vi "(SubVI) Acquire Sinewave True Amplitude A by using Waveform WriteRead_YCC.vi"(5 "f_drive (Hz)":dbl=32.0, 6 "Amplitude, A (nm)":dbl=500.0, 7 "Axis  (Enum)":enum16{"x", "y", "z"}(ring)) -> (1 "True f_drive (Hz)":dbl, 2 "True Amplitude, A (nm)":dbl)   [LabVIEW 2014]
uses:
  Main-Stage-Based/(Global) Current handle and LaserPower_YCC.vi
  <vilib>/gmath/NumericalOptimization/Nonlinear Curve Fit LM formula string.vi
  <vilib>/Utility/file.llb/Write To Spreadsheet File (DBL).vi
  <vilib>/gmath/NI_Gmath.lvlib
panel:
  out "size(s) 2":i32
  out "size(s)":i32
  out "Total Need time (s)":dbl format="%.5f"
  in  "Tab Control":enum32{"Command", "True Output", "Fitting"}(tab)
  out "Write XY Graph 2":cluster{dbl[], "Data Array Out to read":dbl[]}(graph)
  out "Read XY Graph":cluster{dbl[], "Data Array Out to read":dbl[]}(graph)
  out "Read XY Graph 2":cluster{dbl[], "Data Array Out to read":dbl[]}[](graph)
  out "best nonlinear fit for cut position":dbl[](array[numeric])
  in  "Save?":bool
  out "A scaling":dbl
  out "Axis":i32
  out "appended array":dbl[](array[numeric])
  out "Real Current Commanded position (um)":dbl format="%0.5f"
  out "Cut-position array":dbl[](array[numeric])
  out "Cut-Time array":dbl[](array[numeric])
  out "Position Array (um)":dbl[](array[numeric])
  out "Time Array (s)":dbl[](array[numeric])
  out "Sampling Rate (Hz)":dbl
  out "best fit parameters":dbl[](array[numeric])
  out "Read True Position Array (um)":dbl[](array[numeric]) format="%.2f"
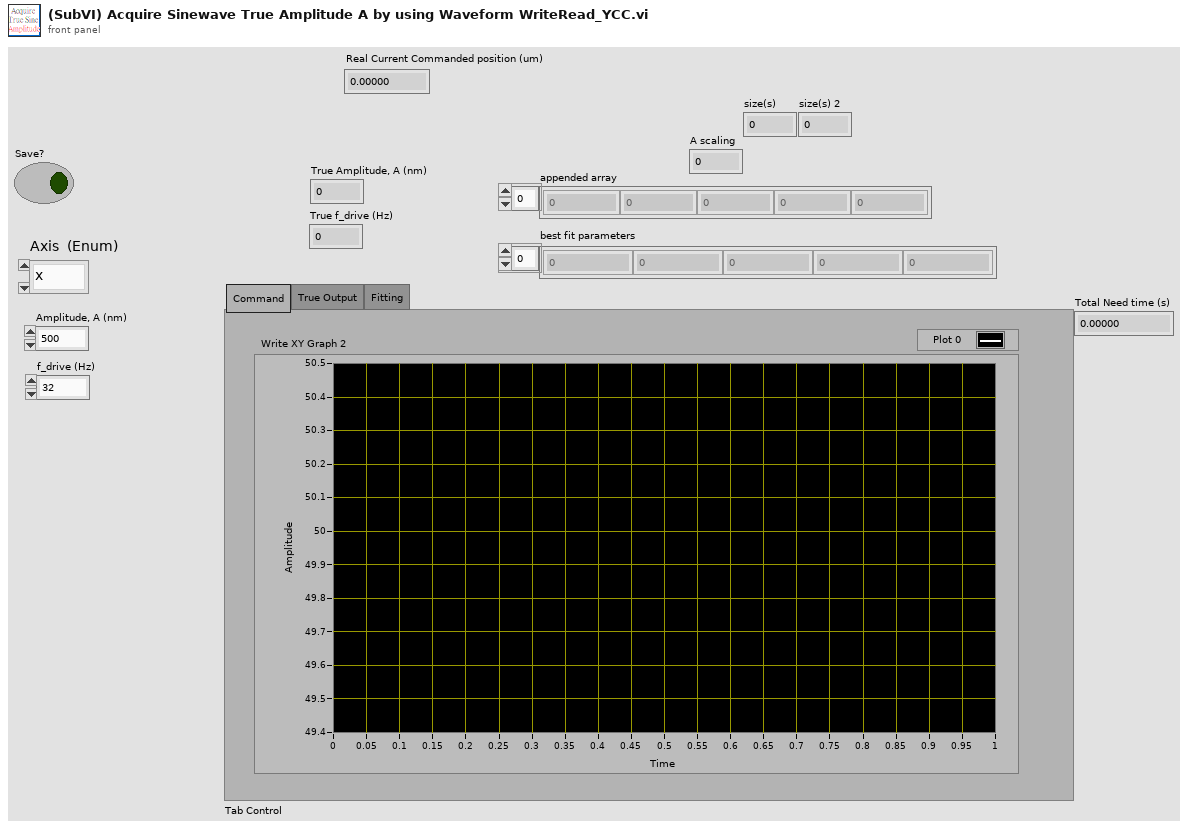
[diagram p1: front panel]
types:
  T1 = enum16{"50 Hz", "60 Hz", "100 Hz", "500 Hz", "1000 Hz", "2000 Hz", "3750 Hz"}
  T2 = cluster{"model":string, "Parameters":string[], "x":string}
  T3 = cluster{"Time Array (s)":dbl[], "Position Array (um)":dbl[]}
  T4 = cluster{"Cut-Time array":dbl[], "best nonlinear fit":dbl[]}
  T5 = cluster{"Cut-Time array":dbl[], "Cut-position array":dbl[]}
  T6 = cluster{"Cut-Time array":dbl[], "Cut-position array":dbl[]}[]
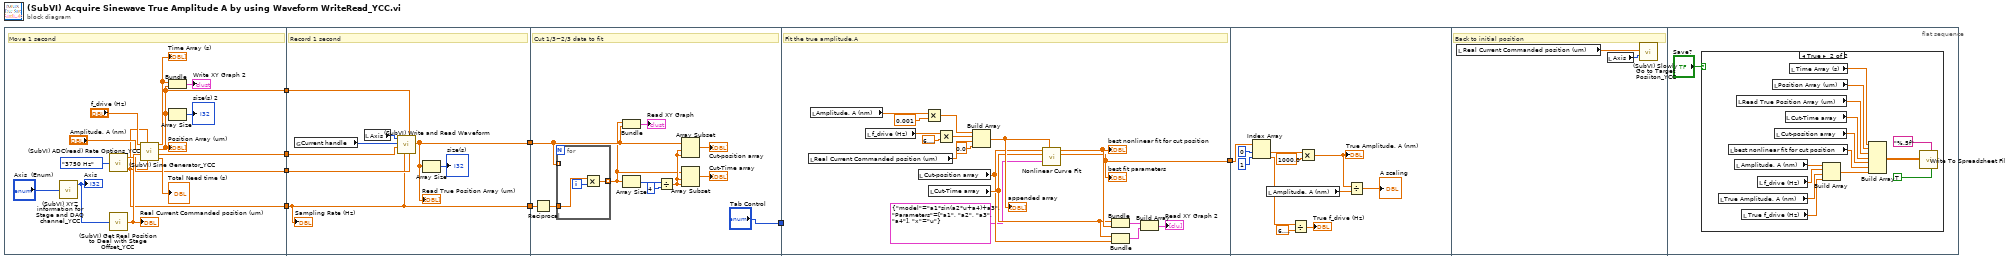
[diagram p0: block diagram]
diagram:
  n1 = flat-sequence {
    tunnel: [w17] -> w8
    tunnel: [w13] -> w7
    tunnel: [w10] -> w3
    tunnel: [w9] -> w2
    tunnel: w8 -> [w28]
    tunnel: w7 -> [w27]
    tunnel: [w26] -> w6
    tunnel: [w23] -> w4
    tunnel: w3 -> [w24]
    tunnel: w2 -> [w23]
    tunnel: w6 -> [w35]
    tunnel: w4 -> [w34]
    tunnel: ["Tab Control"] -> w1
    tunnel: [w54] -> w5
    tunnel: w1 -> [_]
    tunnel: w5 -> [w72]
    frame #0 {
      # "Move 1 second"
      n2 = call "(SubVI) XYZ information for Stage and DAQ channel_YCC.vi"("Axis  (Enum)"="Axis  (Enum)") -> ("Axis"=w15:i32)  [unwired: 3 in, 1 out]
      "Axis" <- w15
      n3 = call "(SubVI) ADC(read) Rate Options_YCC.vi"("ADC Rate for 20bit (ms)"=T1."3750 Hz") -> ("Sampling Rate for reading (Hz)"=w9:dbl, "waiting code for Reading (20bits)"=w10:dbl)  [unwired: 3 in]
      n4 = call "(SubVI) Get Real Position to Deal with Stage Offset_YCC.vi"("Axis"=w15) -> ("Real Current Commanded position (um)"=w20:dbl)  [unwired: 3 in, 1 out]
      "Real Current Commanded position (um)" <- w20
      n5 = call "(SubVI) Sine Generator_YCC.vi"("Points to be generated"=w9, "fs (Hz)"=w9, "initial position (um)"=w20, "Amplitude, A (nm)"="Amplitude, A (nm)", "f_drive (Hz)"="f_drive (Hz)") -> ("Total Need time (s)"=→"Total Need time (s)":dbl, "waiting time (to write) (ms)"=w17:dbl, "Position Array (um)"=w13:dbl[], "Time Array (s)"=w19:dbl[])  [unwired: 1 in]
      "Time Array (s)" <- w19
      "Position Array (um)" <- w13
      n6 = Bundle("Time Array (s)"=w19, "Position Array (um)"=w13) -> (→"Write XY Graph 2":T3)  [unwired: 1 in]
      n7 = Array Size(array=w13) -> (size(s)=→"size(s) 2":i32)
    }
    frame #1 {
      # "Record 1 second"
      n8 = global read "(Global) Current handle and LaserPower_YCC.vi" "Current handle"() -> (w30:i32)
      n9 = local read "Axis"() -> (w29:i32)
      n10 = call "(SubVI) Write and Read Waveform.vi"("ADC Rate (Read)(ms)"=w24, "Data Array In to write"=w27, "Number of Positions to Read"=w23, "DAC Rate (Write) (ms)"=w28, "handle"=w30, "Axis"=w29) -> ("Data Array Out to read"=w26:dbl[])  [unwired: 5 in]
      "Read True Position Array (um)" <- w26
      n11 = Array Size(array=w26) -> (size(s)=→"size(s)":i32)
      "Sampling Rate (Hz)" <- w23
    }
    frame #2 {
      # "Cut 1/3~2/3 data to fit"
      n12 = Reciprocal(x=w34) -> (1/x=w33:dbl)
      n13 = for {
        tunnel: w35 -> [_] mode=indexing
        tunnel: w33 -> [w43]
        tunnel: [w42] -> w32 mode=indexing
        i -> [w44]
        n14 = Multiply(x=w43, y=w44) -> (x*y=w42:dbl)
      }
      n15 = Bundle(w32, "Data Array Out to read"=w35) -> (→"Read XY Graph":cluster{dbl[], "Data Array Out to read":dbl[]})  [unwired: 1 in]
      n16 = Array Size(array=w32) -> (size(s)=w40:i32)
      n17 = Divide(x=w40, y=4) -> (x/y=w38:dbl)
      n18 = Array Subset(array=w35, index=w38, length=w38) -> (→"Cut-position array":dbl[])
      n19 = Array Subset(array=w32, index=w38, length=w38) -> (→"Cut-Time array":dbl[])
    }
    frame #3 {
      # "Fit the true amplitude,A"
      n20 = local read "Real Current Commanded position (um)"() -> (w57:dbl)
      n21 = local read "Amplitude, A (nm)"() -> (w53:dbl)
      n22 = local read "f_drive (Hz)"() -> (w47:dbl)
      n23 = local read "Cut-position array"() -> (w49:dbl[])
      n24 = Multiply(x=w53, y=0.001) -> (x*y=w51:dbl)
      n25 = local read "Cut-Time array"() -> (w50:dbl[])
      n26 = Multiply(x=w47, y=6.283185307179586) -> (x*y=w45:dbl)
      n27 = Build Array(w51, w45, w57, 0.0 ("element")) -> (w55:dbl[])
      "appended array" <- w55
      n28 = call-poly <vilib>:"Nonlinear Curve Fit.vi"("Y"=w49, "initial parameters"=w55, "X"=w50, "model description"=T2 {"model"="a1*sin(a2*u+a4)+a3", "Parameters"=["a1", "a2", "a3", "a4"], "x"="u"}) -> ("best nonlinear fit"=w60:dbl[], "best fit parameters"=w54:dbl[])  [unwired: 7 in, 3 out]
      "best fit parameters" <- w54
      "best nonlinear fit for cut position" <- w60
      n29 = Bundle("Cut-Time array"=w50, "best nonlinear fit"=w60) -> (w59:T4)  [unwired: 1 in]
      n30 = Bundle("Cut-Time array"=w50, "Cut-position array"=w49) -> (w58:T5)  [unwired: 1 in]
      n31 = Build Array(w59, w58) -> (→"Read XY Graph 2":T6)
    }
    frame #4 {
      n32 = Index Array(array=w72, index #1=0 ("index"), index #2=1 ("index")) -> (element #1=w66:dbl, element #2=w65:dbl)
      n33 = local read "Amplitude, A (nm)"() -> (w64:dbl)
      n34 = Divide(x=w65, y=6.283185307179586) -> (x/y=→"True f_drive (Hz)":dbl)
      n35 = Multiply(x=w66, y=1000.0) -> (x*y=w63:dbl)
      "True Amplitude, A (nm)" <- w63
      n36 = Divide(x=w63, y=w64) -> (x/y=→"A scaling":dbl)
    }
    frame #5 {
      # "Back to initial position"
      n37 = local read "Real Current Commanded position (um)"() -> (w73:dbl)
      n38 = local read "Axis"() -> (w74:i32)
      n39 = call "(SubVI) Slowly Go to Target Posiiton_YCC.vi"("axis"=w74, "Target position (um)"=w73) -> ()  [unwired: 2 in, 4 out]
    }
    frame #6 {
      n40 = case shown="True" "Save?" {
        frame False {
        }
        frame True {
          n41 = local read "True Amplitude, A (nm)"() -> (w81:dbl)
          n42 = local read "best nonlinear fit for cut position"() -> (w84:dbl[])
          n43 = local read "Amplitude, A (nm)"() -> (w83:dbl)
          n44 = local read "Read True Position Array (um)"() -> (w87:dbl[])
          n45 = local read "True f_drive (Hz)"() -> (w80:dbl)
          n46 = local read "f_drive (Hz)"() -> (w82:dbl)
          n47 = local read "Position Array (um)"() -> (w88:dbl[])
          n48 = local read "Cut-position array"() -> (w85:dbl[])
          n49 = local read "Cut-Time array"() -> (w86:dbl[])
          n50 = local read "Time Array (s)"() -> (w89:dbl[])
          n51 = Build Array(w83, w82, w81, w80) -> (w79:dbl[])
          n52 = Build Array(w89, w88, w87, w86, w85, w84, w79) -> (w78:dbl[][])
          n53 = call-poly <vilib>:"Write To Spreadsheet File.vi"("transpose? (no:F)"=TRUE, "format (%.3f)"="%.5f", "2D data"=w78) -> ()  [unwired: 5 in, 1 out]
        }
      }
    }
  }
